vi "AI Continuous Smart Read.vi"(4 "Max Value":dbl[](array[numeric]), 5 "Sample Rate":dbl=1000.0 min=1000.0 max=30000.0, 6 "Min Value":dbl[](array[numeric]), 7 "Number of Samples":u32=1000, 8 "error in (no error)":errorcluster, 9 "Timeout":i32=-1 min=-1, 10 "Stop?":bool, 11 "Channel Names":tag[](array[tag])) -> (0 "error out":errorcluster, 3 "Values":dbl[][](array[numeric]))   [LabVIEW 2021, in "AI Continuous.lvlib"]
uses:
  <vilib>/myRIO/Instrument Drivers/Onboard IO/AI Continuous/AI Continuous.lvlib
  <vilib>/myRIO/Common/Instrument Driver Framework/Utilities/typedefs/Generic FPGA Reference.ctl
  <vilib>/myRIO/Common/Instrument Driver Framework/ELVIS III v1.0/AI Continuous/typedefs/ELVIS III v1.0 AI Continuous Channels Enum.ctl
  <vilib>/myRIO/Common/Instrument Driver Framework/ELVIS III v1.0/AI Continuous/typedefs/AI Continuous Channels List.ctl
  <vilib>/myRIO/Common/Instrument Driver Framework/Utilities/typedefs/Analog Scaling Constants.ctl
  <vilib>/myRIO/Common/Instrument Driver Framework/Utilities/typedefs/Hardware Version Enum.ctl
  <vilib>/myRIO/Common/Instrument Driver Framework/Utilities/typedefs/myRIO v1.0 Reference.ctl
  <vilib>/myRIO/Common/Instrument Driver Framework/Utilities/typedefs/myRIO Generic Hardware Reference.ctl
  <vilib>/myRIO/Instrument Drivers/Onboard IO/AI Continuous/typedefs/AI Continuous Reference.ctl
  <vilib>/myRIO/Instrument Drivers/Onboard IO/AI Continuous/vis/myRIO AI Continuous Open.xnode
  <vilib>/myRIO/Common/Instrument Driver Framework/ELVIS III v1.0/AI Continuous/vis/ELVIS III v1.1 Open AI (Continuous).vi
  <vilib>/userdefined/High Color/nirio_resource_hc.ctl
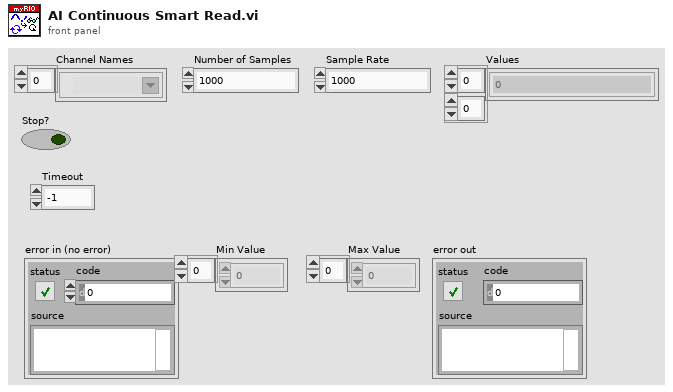
[diagram p1: front panel]
types:
  T1 = typedef "AI Continuous.lvlib/AI Continuous Reference.ctl" = cluster{"myRIO Reference":T2, "AI (Continuous) Channels List":T6, "AI (Continuous) Scaling Constants List":T8[], "Bank Count":u8[]}
  T2 = typedef "myRIO Generic Hardware Reference.ctl" = cluster{"myRIO Model":T3, "myRIO Hardware Reference":T4}
  T3 = typedef "Hardware Version Enum.ctl" = enum16{"Unknown", "myRIO-1900", "myRIO-1950", "roboRIO", "NI ELVIS RIO CM", "ELVIS III"}
  T4 = typedef "myRIO v1.0 Reference.ctl" = cluster{"Generic FPGA Reference":T5, "Allow multiple opens":bool}
  T5 = typedef "Generic FPGA Reference.ctl" = refnum<k20>
  T6 = typedef "AI Continuous Channels List.ctl" = T7[]
  T7 = typedef "ELVIS III v1.0 AI Continuous Channels Enum.ctl" = enum16{"Not Connected", "A/AI0 (Continuous)", "A/AI1 (Continuous)", "A/AI2 (Continuous)", "A/AI3 (Continuous)", "A/AI4 (Continuous)", "A/AI5 (Continuous)", "A/AI6 (Continuous)", "A/AI7 (Continuous)", "A/AI0 (DIFF Continuous)", "A/AI1 (DIFF Continuous)", "A/AI2 (DIFF Continuous)", "A/AI3 (DIFF Continuous)", "B/AI0 (Continuous)", "B/AI1 (Continuous)", "B/AI2 (Continuous)", "B/AI3 (Continuous)", "B/AI4 (Continuous)", "B/AI5 (Continuous)", "B/AI6 (Continuous)", "B/AI7 (Continuous)", "B/AI0 (DIFF Continuous)", "B/AI1 (DIFF Continuous)", "B/AI2 (DIFF Continuous)", "B/AI3 (DIFF Continuous)"}
  T8 = typedef "Analog Scaling Constants.ctl" = cluster{"LSB Weight (Volts)":dbl, "Offset (Volts)":dbl, "Signed?":bool}
  T9 = typedef "nirio_resource_hc.ctl" = tag
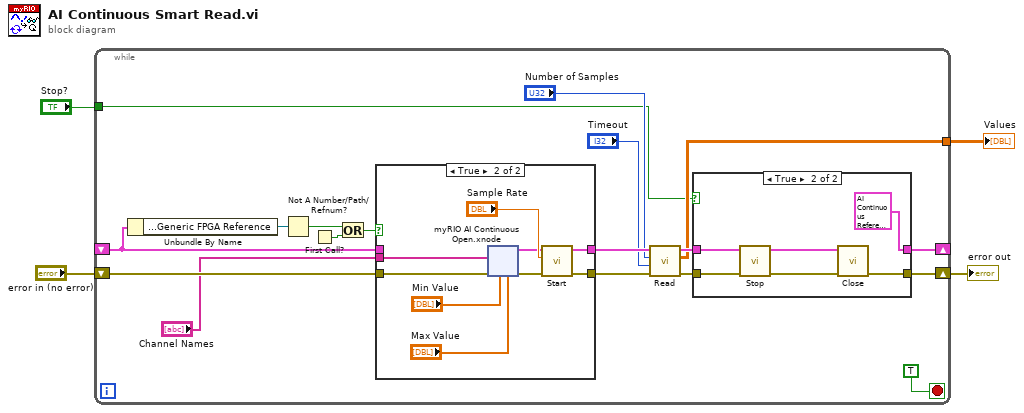
[diagram p0: block diagram]
diagram:
  n1 = while {
    shift-right: [w16] -> w3
    shift-left: "error in (no error)" -> [w19]
    shift-right: [w15] -> _
    shift-left: _ -> [w14]
    tunnel: [w6] -> w2
    tunnel: "Stop?" -> [w5]
    stop <- TRUE stop-if-true
    n2 = Unbundle By Name(w14) -> ("myRIO Reference.myRIO Hardware Reference.Generic FPGA Reference"=w13:T5)
    n3 = Not A Number/Path/Refnum?(number/path/refnum=w13) -> (NaN/Path/Refnum?=w22:bool)
    n4 = First Call?() -> (First Call?: T/F=w21:bool)
    n5 = Or(x=w22, y=w21) -> (x .or. y?=w20:bool)
    n6 = case shown="True" w20 {
      tunnel: w19 -> [w31 w40]
      tunnel: [w31 w33] -> w18
      tunnel: [w32 w35] -> w12
      tunnel: w14 -> [w32 _]
      tunnel: "Channel Names" -> [_ w41]
      frame False {
      }
      frame True {
        n7 = xnode "myRIO AI Continuous Open.xnode"("error in (no error)"=w40, "Channel Names"=w41, "Max Value"="Max Value", "Min Value"="Min Value") -> ("error out"=w34:errorcluster, "AI (Continuous) Ref Out"=w36:T1)
        n8 = call <vilib>:"Start.vi"("error in (no error)"=w34, "Sample Rate"="Sample Rate", "AI (Continuous) Ref In"=w36) -> ("error out"=w33:errorcluster, "AI (Continuous) Ref Out"=w35:T1)  [unwired: 7 in]
      }
    }
    n9 = call <vilib>:"Read.vi"("error in (no error)"=w18, "Timeout"="Timeout", "Number of Samples"="Number of Samples", "AI (Continuous) Ref In"=w12) -> ("error out"=w17:errorcluster, "Values"=w6:dbl[][], "AI (Continuous) Ref Out"=w11:T1)  [unwired: 5 in]
    n10 = case shown="True" w5 {
      tunnel: w17 -> [w24 w30]
      tunnel: [w24 w25] -> w16
      tunnel: [w23 T1 {"myRIO Reference"={"myRIO Model"=enum."Unknown", "myRIO Hardware Reference"={"Generic FPGA Reference"=refnum, "Allow multiple opens"=FALSE}}, "AI (Continuous) Channels List"=[], "AI (Continuous) Scaling Constants List"=[], "Bank Count"=[]} ("AI (Continuous) Ref Out")] -> w15
      tunnel: w11 -> [w23 w29]
      frame False {
      }
      frame True {
        n11 = call <vilib>:"Stop.vi"("error in (no error)"=w30, "AI (Continuous) Ref In"=w29) -> ("error out"=w26:errorcluster, "AI (Continuous) Ref Out"=w27:T1)  [unwired: 8 in]
        n12 = call <vilib>:"Close.vi"("error in (no error)"=w26, "AI (Continuous) Ref In"=w27) -> ("error out"=w25:errorcluster)  [unwired: 9 in]
      }
    }
  }
  "error out" <- w3
  "Values" <- w2
